vi "PassReceiverRole.vi"(6 "Tactic index in":i32, 7 "first call":bool, 8 "error in (no error)":errorcluster, 10 "Game in":refnum<class "Game.lvclass">, 11 "PassReceiverRole in":refnum<class "PassReceiverRole.lvclass">) -> (0 "error out":errorcluster, 1 "tactic index":i32, 2 "Robot out":refnum<class "Robot.lvclass">, 3 "PassReceiverRole out":refnum<class "PassReceiverRole.lvclass">)   [LabVIEW 2024, in "PassReceiverRole.lvclass"]
uses:
  PassReceiverRole.lvclass
  C:/Users/moise/Documents/GitHub/SSL_AI/Role_class/Role.lvclass
  Robot_class/Robot.lvclass
  Game_class/Game.lvclass
  Role_class/Role.lvclass/Role.ctl
  Utilities_class/Utilities.lvclass
  PassReceiverRole.lvclass/PassReceiverRole.ctl
  Tacticbook_class/Tacticbook.lvclass/Tacticbook.ctl
  ShootTactic_class/States.ctl
  ShootTactic_class/ShootTactic.lvclass/ShootTactic.ctl
  Tacticbook_class/Read WaitPassTactic.vi
  Tacticbook_class/Write WaitPassTactic.vi
  Tacticbook_class/Read ShootTactic.vi
  ShootTactic_class/Read States.vi
  Tacticbook_class/Write ShootTactic.vi
  Role_class/Read Tacticbook.vi
  Read number_of_tactics.vi
  Role_class/Write Tacticbook.vi
  Role_class/Write tactic_index.vi
  Role_class/Read RobotRef.vi
  Tacticbook_class/Tacticbook.lvclass
  WaitPassTactic_class/WaitPassTactic.lvclass
  ShootTactic_class/ShootTactic.lvclass
panel:
  out "Game out":refnum<class "Game.lvclass">
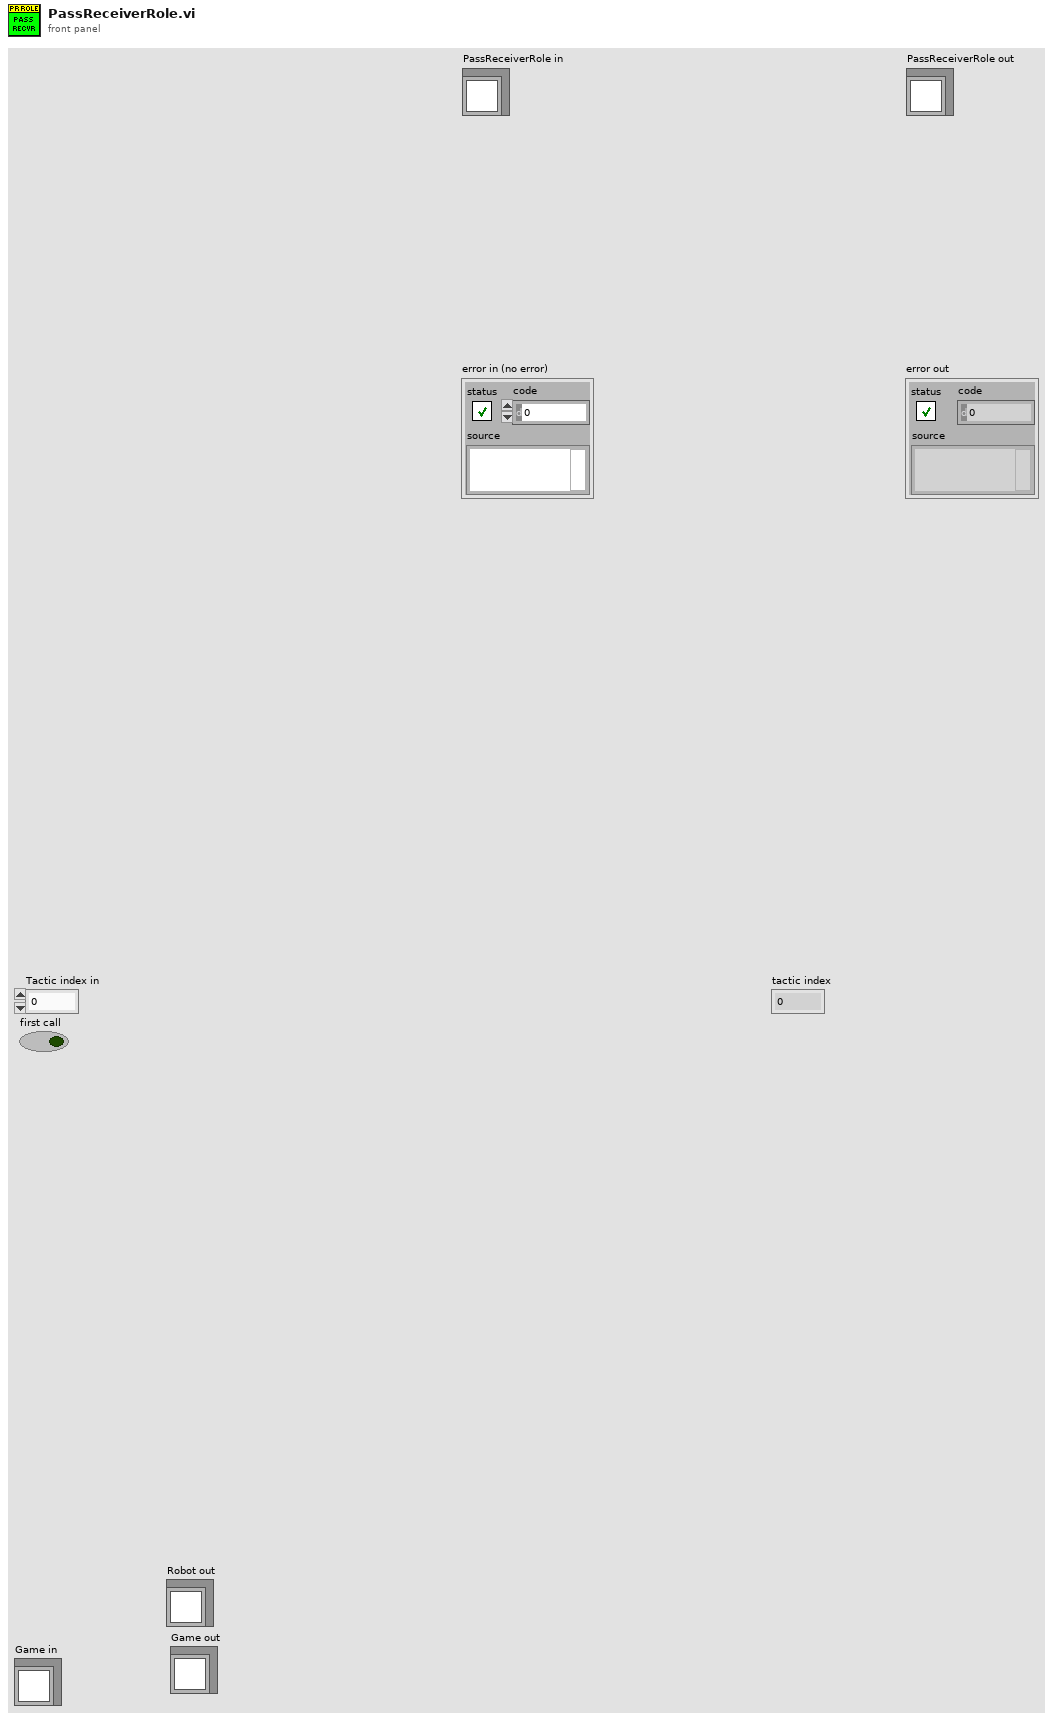
[diagram p1: front panel]
types:
  T1 = typedef "ShootTactic.lvclass/States.ctl" = enum16{"BallInGoalieArea", "Exit", "KickToGoal", "InterceptBall"}
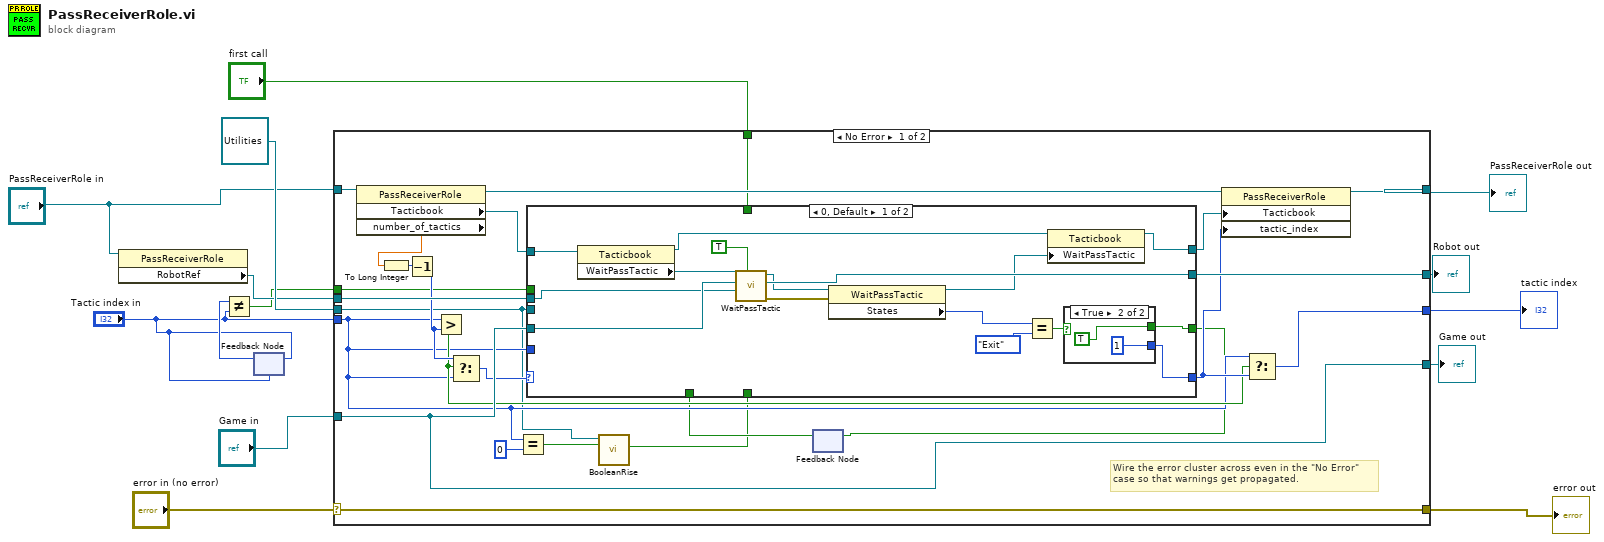
[diagram p0: block diagram]
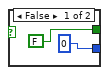
[diagram p2: hidden frame]
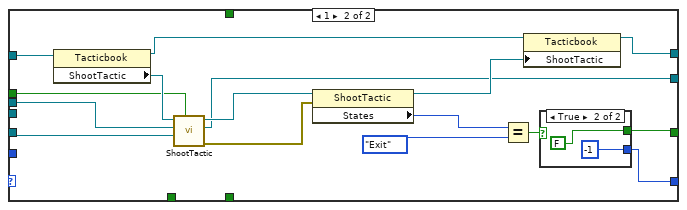
[diagram p3: hidden frame]
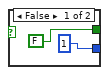
[diagram p4: hidden frame]
diagram:
  n1 = property class="PassReceiverRole"(reference="PassReceiverRole in") -> ("RobotRef"=w5:refnum<class "Robot.lvclass">)  [unwired: 1 in, 2 out]
  n2 = feedback #1("Tactic index in") -> (w3:i32)
  n3 = Not Equal?(x=w3, y="Tactic index in") -> (x != y?=w1:bool)
  n4 = feedback-in #1("Tactic index in") -> ()
  n5 = case shown="No Error" "error in (no error)" {
    selector: "error in (no error)" -> [w39 w83]
    tunnel: [w39 w83] -> w9
    tunnel: [w37 w82] -> w10
    tunnel: "PassReceiverRole in" -> [w38 w82]
    tunnel: w5 -> [w34 w81]
    tunnel: [w33 w81] -> w14
    tunnel: [w31 w80] -> w13
    tunnel: "Game in" -> [w31 w80]
    tunnel: [w26 _] -> w8
    tunnel: "Tactic index in" -> [w25 _]
    tunnel: refnum<class "Utilities.lvclass"> refnum ("Utilities in") -> [w24 _]
    tunnel: "first call" -> [w23 _]
    tunnel: w1 -> [w15 _]
    frame No Error {
      # "Wire the error cluster across even in the \"No Error\"\ncase so that warnings get propagated."
      n6 = property class="PassReceiverRole"(reference=w38) -> (reference out=w36:refnum<class "PassReceiverRole.lvclass">, "Tacticbook"=w35:refnum<class "Tacticbook.lvclass">, "number_of_tactics"=w16:dbl)  [unwired: 1 in, 1 out]
      n7 = To Long Integer(number=w16) -> (32bit integer=w17:i32)
      n8 = Decrement(x=w17) -> (x-1=w30:i32)
      n9 = Greater?(x=w25, y=w30) -> (0:w27:bool)
      n10 = Select(t=w30, s=w27, f=w25) -> (s? t:f=w29:i32)
      n11 = Equal?(x=w25, y=0) -> (x = y?=w20:bool)
      n12 = call "BooleanRise.vi"("Boolean in"=w20, "Utilities in"=w24) -> ("Boolean"=w18:bool)  [unwired: 7 in, 2 out]
      n13 = feedback #2() -> (w21:bool)  [unwired: 1 in]
      n14 = case shown="0, Default" w29 {
        tunnel: [w43 w62] -> w28
        tunnel: w35 -> [w55 w71]
        tunnel: w34 -> [w46 w66]
        tunnel: [w54 w68] -> w33
        tunnel: [w50 w67] -> w32
        tunnel: w31 -> [w47 w65]
        tunnel: w25 -> [_ _]
        tunnel: w24 -> [_ _]
        tunnel: w23 -> [_ _]
        tunnel: [w42 w63] -> w22
        tunnel: w21 -> [_ _]
        tunnel: w18 -> [_ _]
        tunnel: w15 -> [_ w60]
        frame 0, Default {
          n15 = property class="Tacticbook"(reference=w55) -> (reference out=w52:refnum<class "Tacticbook.lvclass">, "WaitPassTactic"=w49:refnum<class "WaitPassTactic.lvclass">)  [unwired: 1 in, 1 out]
          n16 = call-dynamic "WaitPassTactic.vi"("first call"=TRUE, "Robot"=w46, "Game in"=w47, "WaitPassTactic in"=w49) -> ("error out"=w53:errorcluster, "Robot out"=w54:refnum<class "Robot.lvclass">, "WaitPassTactic out"=w48:refnum<class "WaitPassTactic.lvclass">)  [unwired: 5 in]
          n17 = property class="WaitPassTactic"(reference=w48, error in=w53) -> (reference out=w51:refnum<class "WaitPassTactic.lvclass">, "States"=w44:enum16{"State 0", "State 1", "State 2", "Exit"})  [unwired: 1 out]
          n18 = Equal?(x=w44, y=enum16{"State 0", "State 1", "State 2", "Exit"}."Exit") -> (x = y?=w45:bool)
          n19 = property class="Tacticbook"(reference=w52, "WaitPassTactic"=w51) -> (reference out=w50:refnum<class "Tacticbook.lvclass">)  [unwired: 1 in, 1 out]
          n20 = case shown="True" w45 {
            tunnel: [0 1] -> w43
            tunnel: [FALSE TRUE] -> w42
            frame False {
            }
            frame True {
            }
          }
        }
        frame 1 {
          n21 = property class="Tacticbook"(reference=w71) -> (reference out=w75:refnum<class "Tacticbook.lvclass">, "ShootTactic"=w70:refnum<class "ShootTactic.lvclass">)  [unwired: 1 in, 1 out]
          n22 = call "ShootTactic.vi"("firstCall?"=w60, "Game in"=w65, "Robot"=w66, "ShootTactic in"=w70) -> ("error out"=w64:errorcluster, "Robot out"=w68:refnum<class "Robot.lvclass">, "ShootTactic out"=w69:refnum<class "ShootTactic.lvclass">)  [unwired: 4 in, 1 out]
          n23 = property class="ShootTactic"(reference=w69, error in=w64) -> (reference out=w74:refnum<class "ShootTactic.lvclass">, "States"=w72:T1)  [unwired: 1 out]
          n24 = Equal?(x=w72, y=States."Exit" ("States")) -> (x = y?=w73:bool)
          n25 = property class="Tacticbook"(reference=w75, "ShootTactic"=w74) -> (reference out=w67:refnum<class "Tacticbook.lvclass">)  [unwired: 1 in, 1 out]
          n26 = case shown="True" w73 {
            tunnel: [1 -1] -> w62
            tunnel: [FALSE FALSE] -> w63
            frame False {
            }
            frame True {
            }
          }
        }
      }
      n27 = feedback-in #2(w22) -> ()
      n28 = property class="PassReceiverRole"(reference=w36, "Tacticbook"=w32, "tactic_index"=w28) -> (reference out=w37:refnum<class "PassReceiverRole.lvclass">)  [unwired: 1 in, 1 out]
      n29 = Select(t=w25, s=w27, f=w28) -> (s? t:f=w26:i32)
    }
    frame Error {
    }
  }
  "error out" <- w9
  "PassReceiverRole out" <- w10
  "Robot out" <- w14
  "Game out" <- w13
  "tactic index" <- w8
